vi "QDInstrument_Example.vi"() -> ()   [LabVIEW 2016]
uses:
  <vilib>/Analysis/baseanly.llb/Mean (DBL).vi
  <vilib>/Analysis/NI_AALBase.lvlib
panel:
  in  "Instrument\nType":i32(ring) items=["PPMS", "VersaLab", "DynaCool", "SVSM"]
  in  "Remote":bool
  in  "IP Address":string="127.0.0.1"
  out "Field\nStatus":i32(ring) items=["MagnetUnknown"=0, "StablePersistent"=1, "WarmingSwitch"=2, "CoolingSwitch"=3, "StableDriven"=4, "Iterating"=5, "Charging"=6, "Discharging"=7, "CurrentError"=8, "MagnetFailure"=15]
  out "Temperature\nStatus":i32(ring) items=["TemperatureUnknown"=0, "Stable"=1, "Tracking"=2, "Near"=5, "Chasing"=6, "Filling"=7, "Standby"=10, "Disabled"=13, "ImpedanceNotFunction"=14, "TempFailure"=15]
  out "Chamber\nStatus":i32(ring) items=["ChamberUnknown"=0, "PurgedAndSealed"=1, "VentedAndSealed"=2, "Sealed"=3, "Purging"=4, "Venting"=5, "PreHiVac"=6, "HighVac"=7, "PumpContinuous"=8, "VentContinuous"=9, "ChamberFailure"=15]
  out "Field":dbl
  out "Measuring":bool
  in  "Delay":dbl=5.0
  in  "WaitForField":bool=TRUE
  in  "WaitForTemperature":bool=TRUE
  out "Temperature":dbl
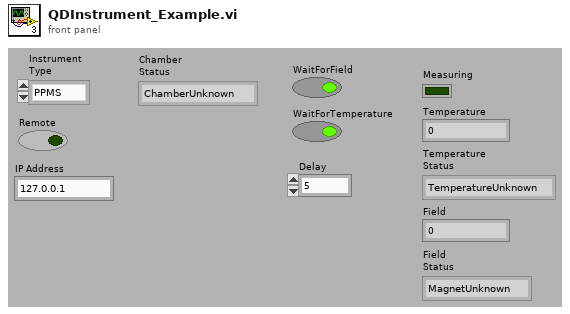
[diagram p1: front panel]
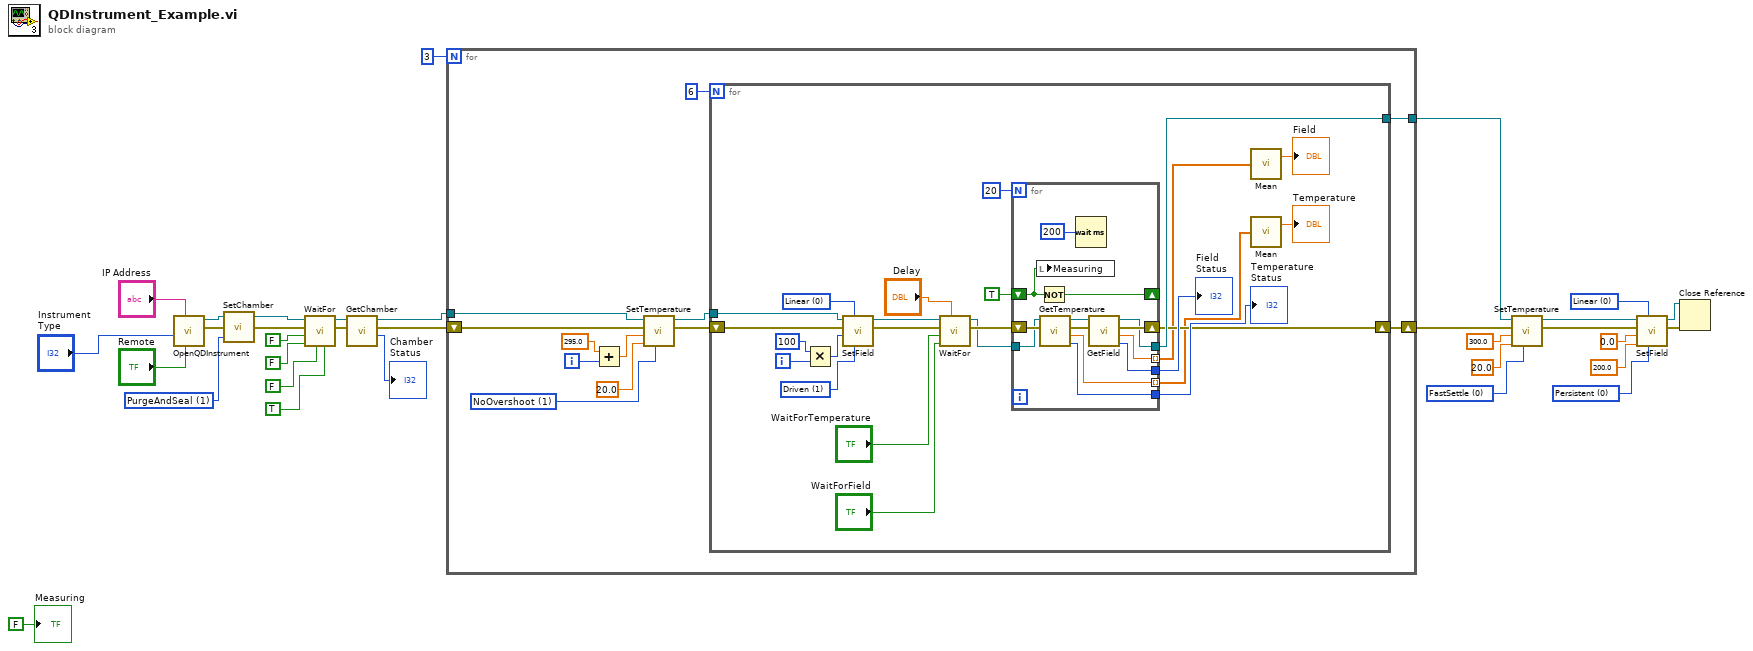
[diagram p0: block diagram]
diagram:
  w29 = 0 items=["Persistent", "Driven"] ("Mode")
  w28 = 0 items=["Linear", "NoOvershoot", "Oscillate"] ("Approach")
  w18 = 1 items=["Seal", "PurgeAndSeal", "VentAndSeal", "PumpContinuous", "VentContinuous", "HighVacuum"] ("Code")
  w9 = 0 items=["FastSettle", "NoOvershoot"] ("Approach")
  n1 = call "OpenQDInstrument.vi"("Remote"="Remote", "IP Address"="IP Address", "Instrument Type"="Instrument\nType") -> ("error out"=w14:errorcluster, "Instrument Ref"=w32:refnum<k24>)  [unwired: 5 in]
  n2 = call "SetChamber.vi"("Code"=w18, "error in (no error)"=w14, "Instrument Ref In"=w32) -> ("error out"=w15:errorcluster, "Instrument Ref Out"=w11:refnum<k24>)  [unwired: 1 out]
  n3 = call "WaitFor.vi"("Wait For Chamber"=TRUE ("WaitForChamber"), "Wait For Position"=FALSE ("WaitForPosition"), "Wait For Field"=FALSE ("WaitForField"), "Wait For Temperature"=FALSE ("WaitForTemperature"), "error in (no error)"=w15, "Instrument Ref In"=w11) -> ("error out"=w16:errorcluster, "Instrument Ref Out"=w12:refnum<k24>)  [unwired: 4 in]
  n4 = call "GetChamber.vi"("error in (no error)"=w16, "Instrument Ref In"=w12) -> ("Chamber\nStatus"=→"Chamber\nStatus":i32, "error out"=w17:errorcluster, "Instrument Ref Out"=w13:refnum<k24>)  [unwired: 2 in, 1 out]
  n5 = for {
    N: 3 -> [_]
    shift-right: [w36] -> w8
    shift-left: w17 -> [w40]
    tunnel: w13 -> [w39]
    tunnel: [w33] -> w4
    i -> [w44]
    w34 = 1 items=["FastSettle", "NoOvershoot"] ("Approach")
    n6 = Add(x=295.0, y=w44) -> (x+y=w42:dbl)
    n7 = call "SetTemperature.vi"("Approach"=w34, "Rate"=20.0, "Temperature"=w42, "error in (no error)"=w40, "Instrument Ref In"=w39) -> ("error out"=w37:errorcluster, "Instrument Ref Out"=w38:refnum<k24>)  [unwired: 2 in, 1 out]
    n8 = for {
      N: 6 -> [_]
      tunnel: w38 -> [w61]
      shift-right: [w50] -> w36
      shift-left: w37 -> [w60]
      tunnel: [w53] -> w33
      i -> [w67]
      w65 = 0 items=["Linear", "NoOvershoot", "Oscillate"] ("Approach")
      w66 = 1 items=["Persistent", "Driven"] ("Mode")
      n9 = Multiply(x=100, y=w67) -> (x*y=w45:i32)
      n10 = call "SetField.vi"("Mode"=w66, "Approach"=w65, "Field"=w45, "error in (no error)"=w60, "Instrument Ref In"=w61) -> ("error out"=w59:errorcluster, "Instrument Ref Out"=w55:refnum<k24>)  [unwired: 2 in, 1 out]
      n11 = call "WaitFor.vi"("Delay"="Delay", "Wait For Field"="WaitForField", "Wait For Temperature"="WaitForTemperature", "error in (no error)"=w59, "Instrument Ref In"=w55) -> ("error out"=w64:errorcluster, "Instrument Ref Out"=w54:refnum<k24>)  [unwired: 5 in]
      n12 = for {
        N: 20 -> [_]
        shift-right: [w81] -> _
        shift-left: TRUE -> [w79]
        shift-right: [w76] -> w50
        shift-left: w64 -> [w78]
        tunnel: w54 -> [w75]
        tunnel: [w73] -> w53
        tunnel: [w70] -> w52
        tunnel: [w69] -> w51
        tunnel: [w71] -> w48 mode=indexing
        tunnel: [w72] -> w49 mode=indexing
        n13 = local write "Measuring"(w79) -> ()
        n14 = Not(x=w79) -> (.not. x?=w81:bool)
        n15 = call "GetTemperature.vi"("error in (no error)"=w78, "Instrument Ref In"=w75) -> ("Temperature\nStatus"=w69:i32, "Temperature"=w72:dbl, "error out"=w77:errorcluster, "Instrument Ref Out"=w74:refnum<k24>)  [unwired: 3 in, 1 out]
        n16 = Wait (ms)(milliseconds to wait=u32 200) -> ()  [unwired: 1 out]
        n17 = call "GetField.vi"("error in (no error)"=w77, "Instrument Ref In"=w74) -> ("Field\nStatus"=w70:i32, "Field"=w71:dbl, "error out"=w76:errorcluster, "Instrument Ref Out"=w73:refnum<k24>)  [unwired: 3 in, 1 out]
      }
      "Field\nStatus" <- w52
      "Temperature\nStatus" <- w51
      n18 = call-poly <vilib>:"Mean.vi"("X"=w48) -> ("mean"=→"Field":dbl)  [unwired: 1 out]
      n19 = call-poly <vilib>:"Mean.vi"("X"=w49) -> ("mean"=→"Temperature":dbl)  [unwired: 1 out]
    }
  }
  n20 = call "SetTemperature.vi"("Approach"=w9, "Rate"=20.0, "Temperature"=300.0, "error in (no error)"=w8, "Instrument Ref In"=w4) -> ("error out"=w25:errorcluster, "Instrument Ref Out"=w24:refnum<k24>)  [unwired: 2 in, 1 out]
  n21 = call "SetField.vi"("Mode"=w29, "Approach"=w28, "Rate"=200.0, "Field"=0.0, "error in (no error)"=w25, "Instrument Ref In"=w24) -> ("error out"=w31:errorcluster, "Instrument Ref Out"=w30:refnum<k24>)  [unwired: 1 in, 1 out]
  n22 = Close Reference(reference=w30, error in (no error)=w31) -> ()  [unwired: 1 out]
  "Measuring" <- FALSE
